vi "createto file(SubVI).vi"(10 "file path (use dialog) in":path, 11 "Array":u32[](array[numeric])) -> ()   [LabVIEW 2015]
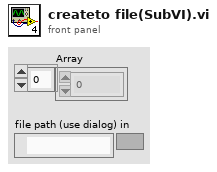
[diagram p1: front panel]
types:
  T1 = enum16{"open", "replace", "create", "open or create", "replace or create", "replace or create with confirmation"}
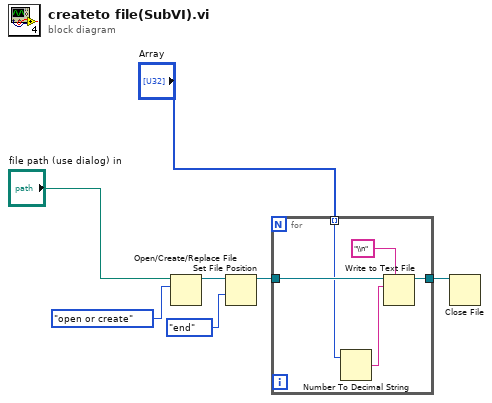
[diagram p0: block diagram]
diagram:
  n1 = Open/Create/Replace File(file path (use dialog)="file path (use dialog) in", operation (0:open)=T1."open or create") -> (refnum out=w4:refnum<file>)  [unwired: 4 in, 2 out]
  n2 = Set File Position(refnum=w4, from (0:start)=enum16{"start", "end", "current"}."end") -> (refnum out=w1:refnum<file>)  [unwired: 2 in, 1 out]
  n3 = for {
    tunnel: w1 -> [w12]
    tunnel: [w11] -> w6
    tunnel: "Array" -> [w9] mode=indexing
    n4 = Number To Decimal String(number=w9) -> (decimal integer string=w10:string)  [unwired: 1 in]
    n5 = Write to Text File(prompt (Choose or enter file path)="\\n", file (use dialog)=w12, text=w10) -> (refnum out=w11:refnum<file>)  [unwired: 1 in, 2 out]
  }
  n6 = Close File(refnum=w6) -> ()  [unwired: 1 in, 2 out]
